vi "Configure Trace Buffer.vi"(5 "Trace Time Rule (1: Absolute)":i32(ring)=1 items=["Delta", "Absolute"], 6 "Trace Buffer Size (100000)":i32=100000, 7 "Trace Buffer Control (1: Never)":i32(ring)=1 items=["Next", "Never"], 8 "error in (no error)":errorcluster, 9 "Trace Buffer Data (2: Sense)":i32(ring)=2 items=["Limit", "Math", "Sense"], 10 "Channel (1: Channel 1)":i32(ring)=1 items=["Channel 1"=1, "Channel 2"=2], 11 "VISA resource name":refnum<visa-resource-name>) -> (0 "error out":errorcluster, 3 "VISA resource name out":refnum<visa-resource-name>)   [LabVIEW 2012, in "Keysight B2980 Series.lvlib"]
doc: "Configures the settings of trace buffer."
uses:
  Keysight B2980 Series.lvlib
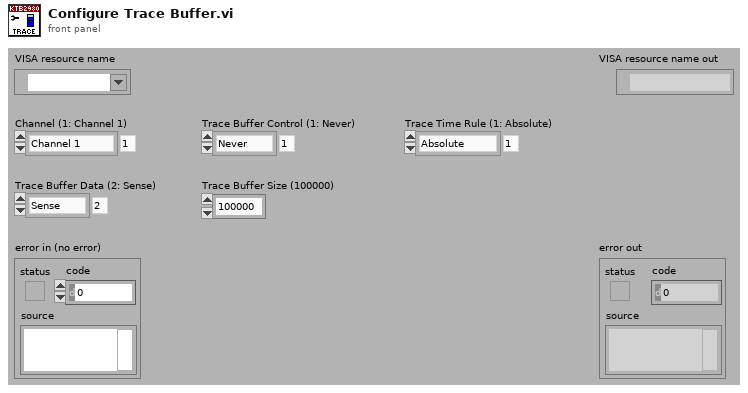
[diagram p1: front panel]
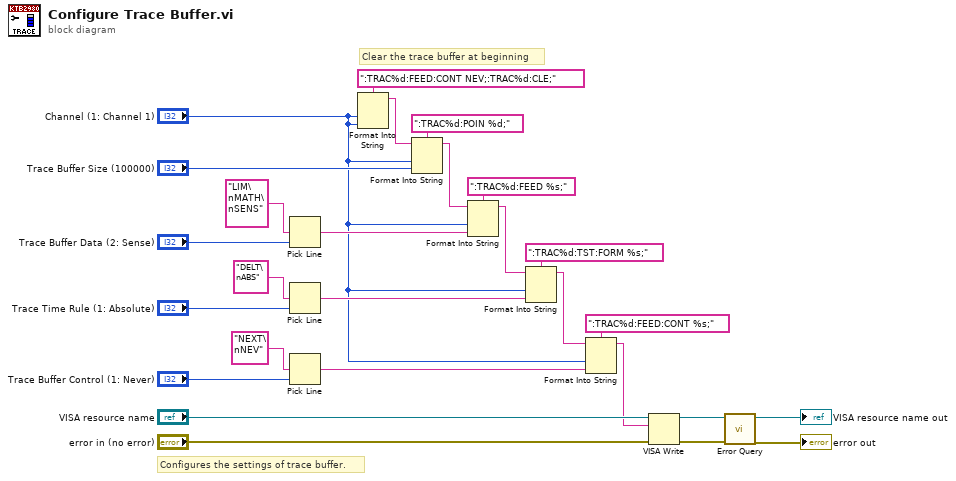
[diagram p0: block diagram]
diagram:
  # "Clear the trace buffer at beginning"
  # "Configures the settings of trace buffer."
  n1 = Pick Line(multi-line string="LIM\nMATH\nSENS", line index="Trace Buffer Data (2: Sense)") -> (output string=w23:string)  [unwired: 1 out]
  n2 = Pick Line(multi-line string="DELT\nABS", line index="Trace Time Rule (1: Absolute)") -> (output string=w13:string)  [unwired: 1 out]
  n3 = Pick Line(multi-line string="NEXT\nNEV", line index="Trace Buffer Control (1: Never)") -> (output string=w19:string)  [unwired: 1 out]
  n4 = Format Into String(format string=":TRAC%d:FEED:CONT NEV;:TRAC%d:CLE;", "Channel (1: Channel 1)", "Channel (1: Channel 1)") -> (resulting string=w8:string)  [unwired: 2 in, 1 out]
  n5 = Format Into String(format string=":TRAC%d:POIN %d;", initial string=w8, "Channel (1: Channel 1)", "Trace Buffer Size (100000)") -> (resulting string=w7:string)  [unwired: 1 in, 1 out]
  n6 = Format Into String(format string=":TRAC%d:FEED %s;", initial string=w7, "Channel (1: Channel 1)", w23) -> (resulting string=w6:string)  [unwired: 1 in, 1 out]
  n7 = Format Into String(format string=":TRAC%d:TST:FORM %s;", initial string=w6, "Channel (1: Channel 1)", w13) -> (resulting string=w5:string)  [unwired: 1 in, 1 out]
  n8 = Format Into String(format string=":TRAC%d:FEED:CONT %s;", initial string=w5, "Channel (1: Channel 1)", w19) -> (resulting string=w1:string)  [unwired: 1 in, 1 out]
  n9 = VISA Write(VISA resource name="VISA resource name", write buffer=w1, error in (no error)="error in (no error)") -> (VISA resource name out=w3:refnum<visa-resource-name>, error out=w2:errorcluster)  [unwired: 1 out]
  n10 = call "Error Query.vi"("error in (no error)"=w2, "VISA resource name"=w3) -> ("error out"=→"error out":errorcluster, "VISA resource name out"=→"VISA resource name out":refnum<visa-resource-name>)  [unwired: 8 out]
